vi "Make New Section if Doesn't Exist.vi"(8 "error in":errorcluster, 9 "Data Folder GUID":string, 10 "Section Name":string, 11 "Parent Section":T1) -> (0 "error out":errorcluster, 3 "New Section":refnum<k24>)   [LabVIEW 2017, in "GE_RM_System Explorer.lvlib"]
uses:
  GE_RM_System Explorer.lvlib
  NationalInstruments.VeriStand.SystemStorage
  <vilib>/NI Veristand/Custom Device API/Custom Device Pointer.ctl
  <vilib>/NI Veristand/Custom Device API/Custom Device API.lvlib
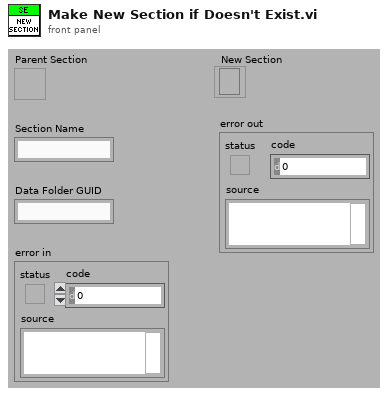
[diagram p1: front panel]
types:
  T1 = typedef "Custom Device API.lvlib/Custom Device Pointer.ctl" = refnum<k24>
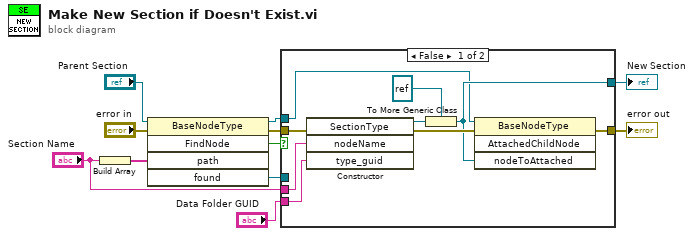
[diagram p0: block diagram]
diagram:
  n1 = Build Array("Section Name") -> (w6:string[])
  n2 = invoke class="BaseNodeType" method="FindNode"(reference="Parent Section", error in="error in", "path"=w6) -> (reference out=w1:T1, error out=w7:errorcluster, "FindNode"=w4:bool, "found"=w2:refnum<k24>)  [unwired: 2 in, 1 out]
  n3 = case shown="False" w4 {
    tunnel: "Data Folder GUID" -> [w17 _]
    tunnel: "Section Name" -> [w16 _]
    tunnel: w7 -> [w15 w21]
    tunnel: [w14 w21] -> w10
    tunnel: [w13 w22] -> w3
    tunnel: w2 -> [_ w22]
    tunnel: w1 -> [w12 _]
    frame False {
      n4 = constructor class="SectionType"(error in=w15, "nodeName"=w16, "type_guid"=w17) -> (reference out=w18:refnum<k24>, error out=w19:errorcluster)  [unwired: 2 in, 3 out]
      n5 = To More Generic Class(target class=refnum<k24> refnum, reference=w18) -> (generic class reference=w13:refnum<k24>)
      n6 = invoke class="BaseNodeType" method="AttachedChildNode"(reference=w12, error in=w19, "nodeToAttached"=w13) -> (error out=w14:errorcluster)  [unwired: 1 in, 3 out]
    }
    frame True {
    }
  }
  "error out" <- w10
  "New Section" <- w3
